vi "Renishaw-XL80_Reinitialize.vi"(8 "error in (no error)":errorcluster, 11 "Renishaw-XL80 in":refnum<class "Renishaw-XL80.lvclass">) -> (0 "error out":errorcluster, 1 "Serial Number":string, 2 "Connect":bool, 3 "Renishaw-XL80 out":refnum<class "Renishaw-XL80.lvclass">)   [LabVIEW 2024, in "Renishaw-XL80.lvclass"]
uses:
  Renishaw-XL80.lvclass
  Renishaw-XL80.lvclass/Renishaw-XL80.ctl
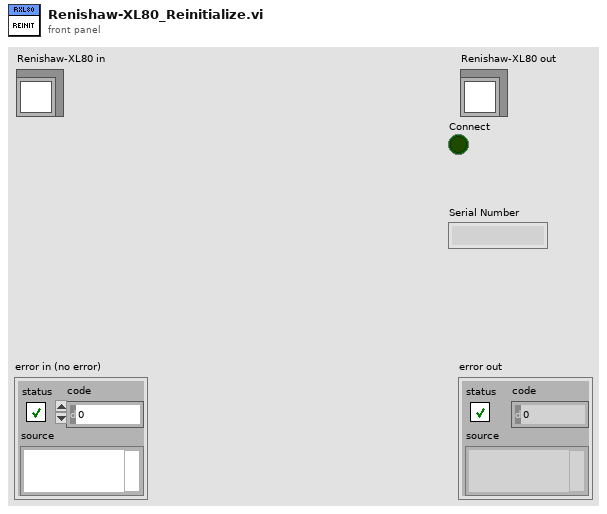
[diagram p1: front panel]
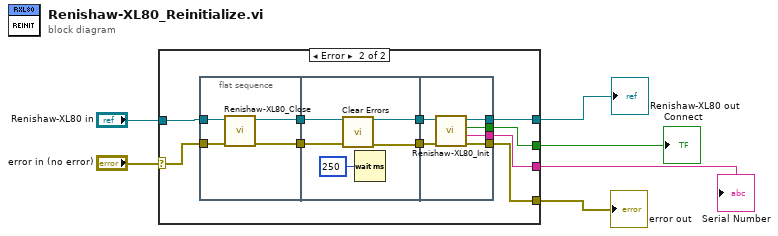
[diagram p0: block diagram]
diagram:
  n1 = case shown="Error" "error in (no error)" {
    selector: "error in (no error)" -> [w8 w18]
    tunnel: [w8 w17] -> w5
    tunnel: [w7 w15] -> w3
    tunnel: "Renishaw-XL80 in" -> [w7 w16]
    tunnel: [_ w10] -> w2
    tunnel: [_ w9] -> w1
    frame No Error {
    }
    frame Error {
      n2 = flat-sequence {
        tunnel: w16 -> [w22]
        tunnel: w18 -> [w20]
        tunnel: [w21] -> w14
        tunnel: [w19] -> w13
        tunnel: w14 -> [w26]
        tunnel: w13 -> [w24]
        tunnel: [w26] -> w12
        tunnel: [w23] -> w11
        tunnel: w12 -> [w31]
        tunnel: w11 -> [w32]
        tunnel: [w30] -> w17
        tunnel: [w29] -> w15
        tunnel: [w28] -> w10
        tunnel: [w27] -> w9
        frame #0 {
          n3 = call-dynamic "Renishaw-XL80_Close.vi"("error in (no error)"=w20, "Renishaw-XL80 in"=w22) -> ("error out"=w19:errorcluster, "Renishaw-XL80 out"=w21:refnum<class "Renishaw-XL80.lvclass">)  [unwired: 8 in]
        }
        frame #1 {
          n4 = call <vilib>:"Clear Errors.vi"("error in (no error)"=w24) -> ("error out"=w23:errorcluster)  [unwired: 5 in, 1 out]
          n5 = Wait (ms)(milliseconds to wait=u32 250) -> ()  [unwired: 1 out]
        }
        frame #2 {
          n6 = call-dynamic "Renishaw-XL80_Init.vi"("error in (no error)"=w32, "Renishaw-XL80 in"=w31) -> ("error out"=w30:errorcluster, "Serial Number"=w27:string, "Connect"=w28:bool, "Renishaw-XL80 out"=w29:refnum<class "Renishaw-XL80.lvclass">)  [unwired: 6 in]
        }
      }
    }
  }
  "error out" <- w5
  "Renishaw-XL80 out" <- w3
  "Connect" <- w2
  "Serial Number" <- w1
